vi "SelectMenu.vi"(0 "XRef":T12, 1 "Tag":T7, 2 "Point":T10, 3 "Menu Type":T9, 4 "State In":T1) -> (14 "Reply":T6, 15 "Handled?":T8, 16 "Multi Object Popup Options":T5, 17 "Fatal Error Out":T4, 18 "State Out":T1)   [LabVIEW 2018, in "RetryNode.xnode"]
uses:
  RetryNode.xnode
  <vilib>/XNodeSupport/XNodeXNodeRef.ctl
  <vilib>/XNodeSupport/XNodeString.ctl
  <vilib>/XNodeSupport/XNodePoint.ctl
  <vilib>/XNodeSupport/XNodeInt.ctl
  <vilib>/XNodeSupport/XNodeMenuType.ctl
  State.ctl
  <vilib>/Utility/miscctls.llb/LVRectTypeDef.ctl
  Options.ctl
  <vilib>/XNodeSupport/XNodeStringArray.ctl
  <vilib>/XNodeSupport/XNodeBool.ctl
  <vilib>/XNodeSupport/XNodeMultiObjectPopupOptions.ctl
  <vilib>/XNodeSupport/XNodeErrorCluster.ctl
  <vilib>/XNodeSupport/NI_XNodeSupport.lvlib
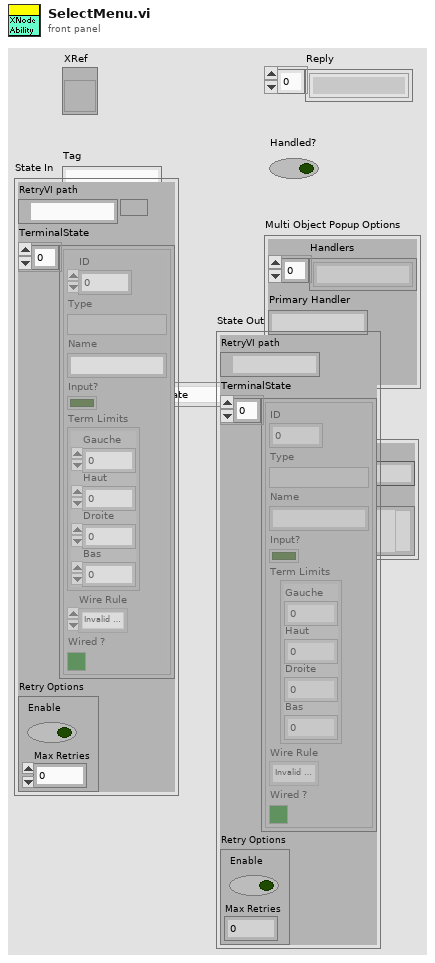
[diagram p1: front panel]
types:
  T1 = typedef "RetryNode.xnode/State.ctl" = cluster{"RetryVI path":path, "TerminalState":cluster{"ID":i32, "Type":variant, "Name":string, "Input?":bool, "Term Limits":T2, "Wire Rule":enum16{"Invalid Wire Rule", "Required", "Recommended", "Optional", "Dynamic Dispatch"}, "Wired ?":bool}[], "Retry Options":T3}
  T2 = typedef "LVRectTypeDef.ctl" = cluster{"Left":i16, "Top":i16, "Right":i16, "Bottom":i16}
  T3 = typedef "RetryNode.xnode/Options.ctl" = cluster{"Enable":bool, "Max Retries":i32}
  T4 = typedef "NI_XNodeSupport.lvlib/XNodeErrorCluster.ctl" = errorcluster
  T5 = typedef "NI_XNodeSupport.lvlib/XNodeMultiObjectPopupOptions.ctl" = cluster{"Handlers":T6, "Primary Handler":T7, "Stop Processing?":T8}
  T6 = typedef "NI_XNodeSupport.lvlib/XNodeStringArray.ctl" = T7[]
  T7 = typedef "NI_XNodeSupport.lvlib/XNodeString.ctl" = string
  T8 = typedef "NI_XNodeSupport.lvlib/XNodeBool.ctl" = bool
  T9 = typedef "NI_XNodeSupport.lvlib/XNodeMenuType.ctl" = enum32{"Single Object Operate", "Single Object Popup", "Multi Object Popup Master", "Multi Object Popup Other"}
  T10 = typedef "NI_XNodeSupport.lvlib/XNodePoint.ctl" = cluster{"H":T11, "V":T11}
  T11 = typedef "NI_XNodeSupport.lvlib/XNodeInt.ctl" = i32
  T12 = typedef "NI_XNodeSupport.lvlib/XNodeXNodeRef.ctl" = refnum<vi>
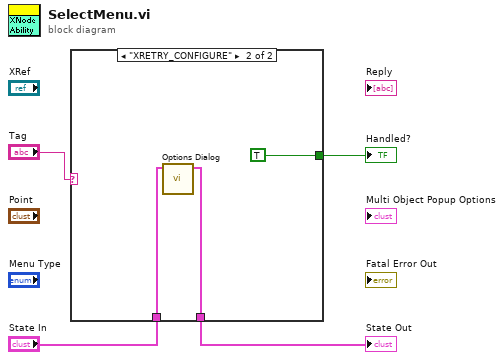
[diagram p0: block diagram]
diagram:
  n1 = case shown="\"XRETRY_CONFIGURE\"" "Tag" {
    tunnel: "State In" -> [w5 w8]
    tunnel: [w5 w7] -> w2
    tunnel: [_ TRUE] -> w1
    frame Default {
    }
    frame "XRETRY_CONFIGURE" {
      n2 = call "Options Dialog.vi"("State In"=w8) -> ("State Out"=w7:T1)  [unwired: 10 in]
    }
  }
  "Handled?" <- w1
  "State Out" <- w2
